vi "OC2 Find start.vi"(9 "input string":string, 11 "Command":string) -> (1 "substring":string)   [LabVIEW 2009]
panel:
  # "Find Start"
  # "V1.02"
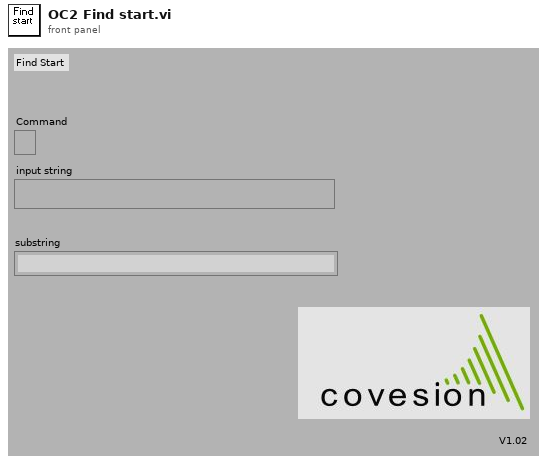
[diagram p1: front panel]
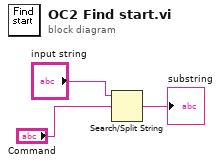
[diagram p0: block diagram]
diagram:
  n1 = Search/Split String(string="input string", search string/char (-)="Command") -> (match + rest of string=→"substring":string)  [unwired: 1 in, 2 out]
